vi "Load Channel Status.vi"(8 "error in (no error)":errorcluster, 11 "S4GUI in":refnum<class "S4GUI.lvclass">) -> (0 "error out":errorcluster, 3 "S4GUI out":refnum<class "S4GUI.lvclass">)   [LabVIEW 2018, in "S4GUI.lvclass"]
uses:
  S4GUI.lvclass
  S4GUI.lvclass/S4GUI.ctl
  Server/Server.lvclass/Server.ctl
  Acquisition/Acquisition.lvclass
  C:/Users/devstaff/sparc4/s4gui/Versao ZeroMQ REQ-REP/SPARC4_GUI -v1.0.0/Server/Server.lvclass
  Channel/Channel.lvclass
  Server/Server.lvclass
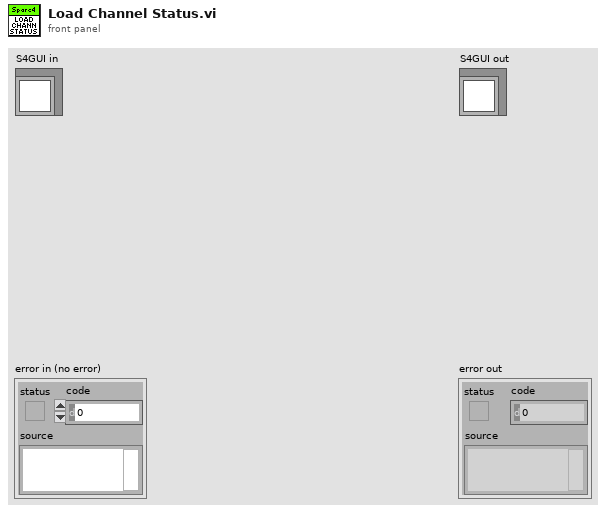
[diagram p1: front panel]
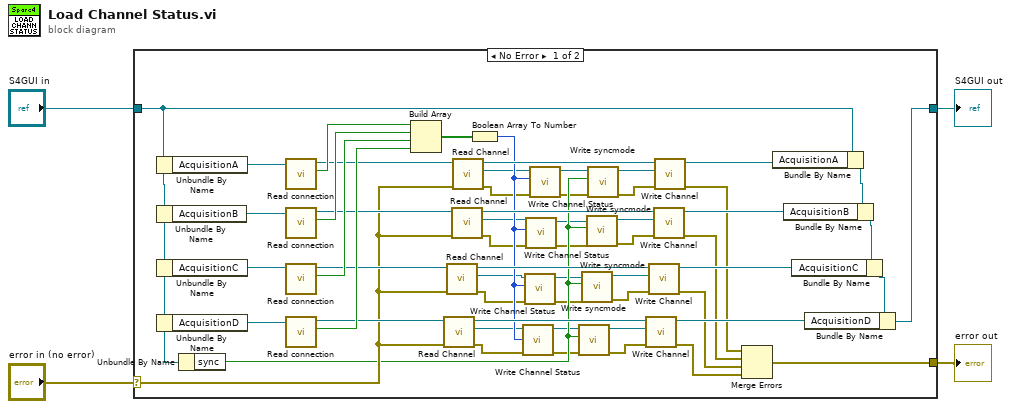
[diagram p0: block diagram]
diagram:
  n1 = case shown="No Error" "error in (no error)" {
    selector: "error in (no error)" -> [w23 w64]
    tunnel: [w24 w64] -> w3
    tunnel: [w49 w63] -> w1
    tunnel: "S4GUI in" -> [w53 w63]
    frame No Error {
      n2 = Unbundle By Name(w53) -> ("AcquisitionA"=w62:refnum<class "Acquisition.lvclass">)
      n3 = Unbundle By Name(w53) -> ("AcquisitionB"=w61:refnum<class "Acquisition.lvclass">)
      n4 = Unbundle By Name(w53) -> ("AcquisitionC"=w60:refnum<class "Acquisition.lvclass">)
      n5 = Unbundle By Name(w53) -> ("AcquisitionD"=w59:refnum<class "Acquisition.lvclass">)
      n6 = Unbundle By Name(w53) -> ("sync"=w22:bool)
      n7 = call "Read connection.vi"("Server in"=w62) -> ("connection"=w58:bool, "Server out"=w48:refnum<class "Acquisition.lvclass">)  [unwired: 8 in, 1 out]
      n8 = call "Read connection.vi"("Server in"=w61) -> ("connection"=w57:bool, "Server out"=w42:refnum<class "Acquisition.lvclass">)  [unwired: 8 in, 1 out]
      n9 = call "Read connection.vi"("Server in"=w60) -> ("connection"=w56:bool, "Server out"=w35:refnum<class "Acquisition.lvclass">)  [unwired: 8 in, 1 out]
      n10 = call "Read connection.vi"("Server in"=w59) -> ("connection"=w55:bool, "Server out"=w33:refnum<class "Acquisition.lvclass">)  [unwired: 8 in, 1 out]
      n11 = Build Array(w58, w57, w56, w55) -> (w54:bool[])
      n12 = call-dynamic "Read Channel.vi"("error in (no error)"=w23, "Acquisition in"=w33) -> ("error out"=w9:errorcluster, "Channel.lvclass"=w14:refnum<class "Channel.lvclass">, "Acquisition out"=w36:refnum<class "Acquisition.lvclass">)  [unwired: 7 in]
      n13 = call-dynamic "Read Channel.vi"("error in (no error)"=w23, "Acquisition in"=w35) -> ("error out"=w10:errorcluster, "Channel.lvclass"=w16:refnum<class "Channel.lvclass">, "Acquisition out"=w38:refnum<class "Acquisition.lvclass">)  [unwired: 7 in]
      n14 = call-dynamic "Read Channel.vi"("error in (no error)"=w23, "Acquisition in"=w42) -> ("error out"=w11:errorcluster, "Channel.lvclass"=w18:refnum<class "Channel.lvclass">, "Acquisition out"=w41:refnum<class "Acquisition.lvclass">)  [unwired: 7 in]
      n15 = call-dynamic "Read Channel.vi"("error in (no error)"=w23, "Acquisition in"=w48) -> ("error out"=w12:errorcluster, "Channel.lvclass"=w20:refnum<class "Channel.lvclass">, "Acquisition out"=w47:refnum<class "Acquisition.lvclass">)  [unwired: 7 in]
      n16 = Boolean Array To Number(Boolean array=w54) -> (number=w21:u32)
      n17 = call-dynamic "Write Channel Status.vi"("error in (no error)"=w9, "Channel Status"=w21, "Channel in"=w14) -> ("error out"=w8:errorcluster, "Channel out"=w13:refnum<class "Channel.lvclass">)  [unwired: 7 in]
      n18 = call-dynamic "Write Channel Status.vi"("error in (no error)"=w10, "Channel Status"=w21, "Channel in"=w16) -> ("error out"=w7:errorcluster, "Channel out"=w15:refnum<class "Channel.lvclass">)  [unwired: 7 in]
      n19 = call-dynamic "Write Channel Status.vi"("error in (no error)"=w11, "Channel Status"=w21, "Channel in"=w18) -> ("error out"=w6:errorcluster, "Channel out"=w17:refnum<class "Channel.lvclass">)  [unwired: 7 in]
      n20 = call-dynamic "Write Channel Status.vi"("error in (no error)"=w12, "Channel Status"=w21, "Channel in"=w20) -> ("error out"=w5:errorcluster, "Channel out"=w19:refnum<class "Channel.lvclass">)  [unwired: 7 in]
      n21 = call-dynamic "Write syncmode.vi"("error in (no error)"=w8, "syncmode"=w22, "Channel in"=w13) -> ("error out"=w37:errorcluster, "Channel out"=w29:refnum<class "Channel.lvclass">)  [unwired: 7 in]
      n22 = call-dynamic "Write syncmode.vi"("error in (no error)"=w7, "syncmode"=w22, "Channel in"=w15) -> ("error out"=w39:errorcluster, "Channel out"=w30:refnum<class "Channel.lvclass">)  [unwired: 7 in]
      n23 = call-dynamic "Write syncmode.vi"("error in (no error)"=w6, "syncmode"=w22, "Channel in"=w17) -> ("error out"=w43:errorcluster, "Channel out"=w31:refnum<class "Channel.lvclass">)  [unwired: 7 in]
      n24 = call-dynamic "Write syncmode.vi"("error in (no error)"=w5, "syncmode"=w22, "Channel in"=w19) -> ("error out"=w44:errorcluster, "Channel out"=w46:refnum<class "Channel.lvclass">)  [unwired: 7 in]
      n25 = call-dynamic "Write Channel.vi"("error in (no error)"=w37, "Channel.lvclass"=w29, "Acquisition in"=w36) -> ("error out"=w25:errorcluster, "Acquisition out"=w32:refnum<class "Acquisition.lvclass">)  [unwired: 7 in]
      n26 = call-dynamic "Write Channel.vi"("error in (no error)"=w39, "Channel.lvclass"=w30, "Acquisition in"=w38) -> ("error out"=w26:errorcluster, "Acquisition out"=w34:refnum<class "Acquisition.lvclass">)  [unwired: 7 in]
      n27 = call-dynamic "Write Channel.vi"("error in (no error)"=w43, "Channel.lvclass"=w31, "Acquisition in"=w41) -> ("error out"=w27:errorcluster, "Acquisition out"=w40:refnum<class "Acquisition.lvclass">)  [unwired: 7 in]
      n28 = call-dynamic "Write Channel.vi"("error in (no error)"=w44, "Channel.lvclass"=w46, "Acquisition in"=w47) -> ("error out"=w28:errorcluster, "Acquisition out"=w45:refnum<class "Acquisition.lvclass">)  [unwired: 7 in]
      n29 = Merge Errors(w28, w27, w26, w25) -> (w24:errorcluster)
      n30 = Bundle By Name(cluster=w53, "AcquisitionA"=w45) -> (w52:refnum<class "S4GUI.lvclass">)
      n31 = Bundle By Name(cluster=w52, "AcquisitionB"=w40) -> (w51:refnum<class "S4GUI.lvclass">)
      n32 = Bundle By Name(cluster=w51, "AcquisitionC"=w34) -> (w50:refnum<class "S4GUI.lvclass">)
      n33 = Bundle By Name(cluster=w50, "AcquisitionD"=w32) -> (w49:refnum<class "S4GUI.lvclass">)
    }
    frame Error {
    }
  }
  "error out" <- w3
  "S4GUI out" <- w1
